vi "readfile.vi"(9 "count":i32=-1, 10 "file (use dialog)":path) -> (0 "channels":dbl[][](array[numeric]), 1 "clipping":dbl[][](array[numeric]), 2 "attenuator":dbl[][](array[numeric]), 3 "voltage":dbl[](array[numeric]), 4 "XY Graph":cluster{dbl[], dbl[]}[](graph), 6 "XY Graph 2":cluster{dbl[], dbl[]}[](graph))   [LabVIEW 2009]
panel:
  in  "file out":string="all"
  in  "file":string="all"
  out "element":i32
  out "Numeric 3":i32
  out "Numeric 2":i32
  out "size(s)":i32[](array[numeric])
  out "subarray 2":dbl[](array[numeric])
  out "Data":dbl[][][](array[numeric])
  out "data":dbl[][](array[numeric])
  out "clipping array":dbl[](array[numeric])
  out "attenuator array":dbl[](array[numeric])
  out "channels array":dbl[](array[numeric])
  out "before substring":string
  out "Numeric":i32
  out "length":i32
  out "cancelled":bool
  in  "prompt (Open existing file)":string
  out "refnum out":refnum<file>
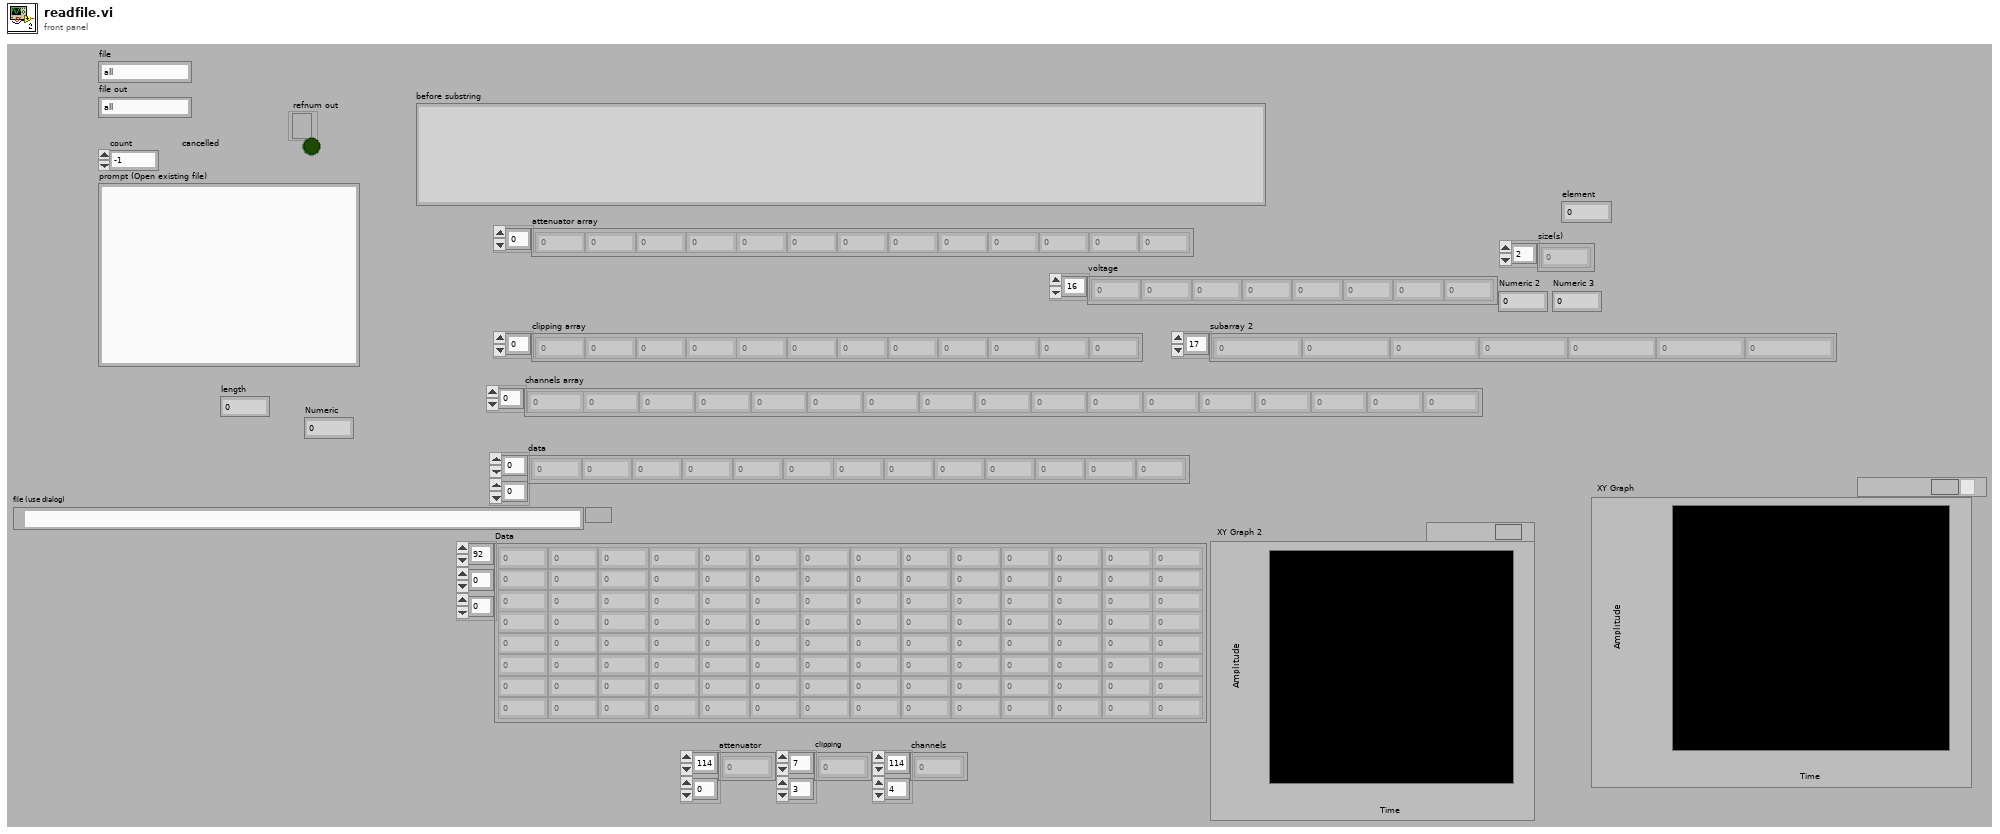
[diagram p1: front panel]
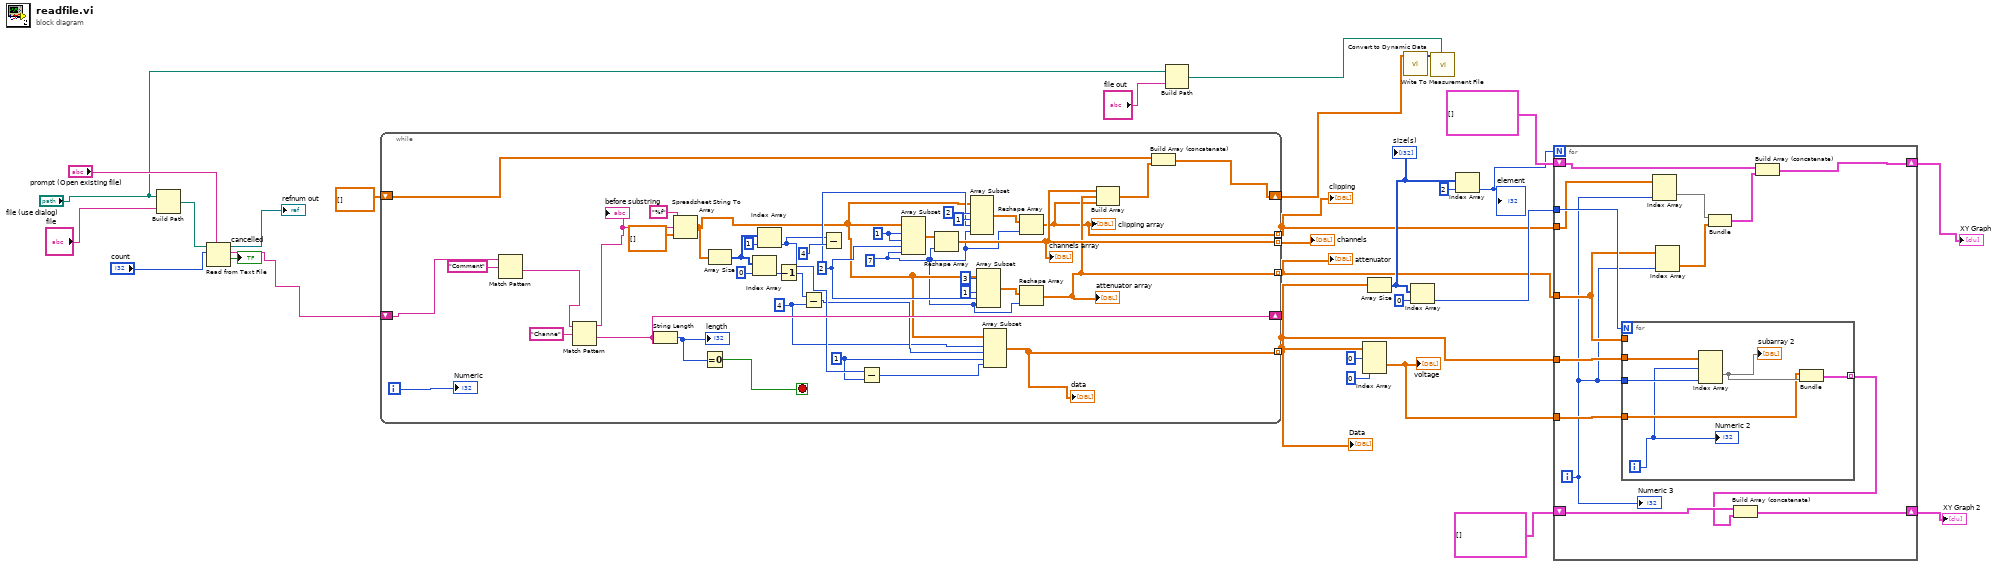
[diagram p0: block diagram]
diagram:
  n1 = Build Path(base path="file (use dialog)", name or relative path="file") -> (appended path=w6:path)
  n2 = Read from Text File(prompt (Open existing file)="prompt (Open existing file)", file (use dialog)=w6, count="count") -> (refnum out=→"refnum out":refnum<file>, text=w25:string, cancelled=→"cancelled":bool)  [unwired: 1 in, 1 out]
  n3 = while {
    shift-right: [w63] -> _
    shift-left: w25 -> [w66]
    tunnel: [w34] -> w9 mode=indexing
    tunnel: [w36] -> w11 mode=indexing
    tunnel: [w37] -> w12 mode=indexing
    tunnel: [w35] -> w10 mode=indexing
    shift-right: [w32] -> w2
    shift-left: dbl[][] [] -> [w31]
    i -> [w67]
    stop <- w68 stop-if-true
    w30 = 7 ("y")
    w38 = 1 ("index")
    w40 = 4 ("y")
    w55 = 1 ("length")
    w52 = 2 ("index")
    n4 = Match Pattern(string=w66, regular expression="Comment") -> (after substring=w64:string)  [unwired: 1 in, 3 out]
    n5 = Match Pattern(string=w64, regular expression="Channe") -> (before substring=w61:string, after substring=w63:string)  [unwired: 1 in, 2 out]
    "before substring" <- w61
    n6 = String Length(string=w63) -> (length=w69:i32)
    "length" <- w69
    n7 = Spreadsheet String To Array(format string="%f", spreadsheet string=w61, array type (2D Dbl)=dbl[][] []) -> (array=w42:dbl[][])  [unwired: 1 in]
    n8 = Equal To 0?(x=w69) -> (x = 0?=w68:bool)
    n9 = Array Size(array=w42) -> (size(s)=w47:i32[])
    n10 = Index Array(array=w47, index=0) -> (element=w44:i32)
    n11 = Index Array(array=w47, index=1) -> (element=w45:i32)
    n12 = Decrement(x=w44) -> (x-1=w43:i32)
    n13 = Subtract(x=w43, y=w40) -> (x-y=w41:i32)
    n14 = Subtract(x=w45, y=4) -> ()  [unwired: 1 out]
    n15 = Subtract(x=w45, y=w38) -> (x-y=w39:i32)
    n16 = Array Subset(array=w42, index (row)=w55, length (row)=w55, index (col)=w52, length (col)=w30) -> (w58:dbl[][])
    n17 = Reshape Array(w58, w30) -> (w36:dbl[])
    "channels array" <- w36
    n18 = Array Subset(array=w42, index (row)=2 ("index"), length (row)=1 ("length"), index (col)=w52, length (col)=w30) -> (w49:dbl[][])
    n19 = Array Subset(array=w42, index (row)=3 ("index"), length (row)=1 ("length"), index (col)=w52, length (col)=w30) -> (w48:dbl[][])
    n20 = Array Subset(array=w42, index (row)=w40, length (row)=w41, index (col)=w38, length (col)=w39) -> (w37:dbl[][])
    "data" <- w37
    n21 = Reshape Array(w49, w30) -> (w34:dbl[])
    "clipping array" <- w34
    n22 = Reshape Array(w48, w30) -> (w35:dbl[])
    "attenuator array" <- w35
    n23 = Build Array(w36, w35, w34) -> (w33:dbl[][])
    n24 = Build Array (concatenate)(w31, w33) -> (w32:dbl[][])
    "Numeric" <- w67
  }
  "Data" <- w12
  "attenuator" <- w10
  "clipping" <- w9
  "channels" <- w11
  n25 = Build Path(base path="file (use dialog)", name or relative path="file out") -> (appended path=w3:path)
  n26 = Index Array(array=w12, index (dim 0)=0 ("disabled index (page)"), index (dim 2)=0 ("disabled index (col)")) -> (element=w22:dbl[])  [unwired: 1 in]
  "voltage" <- w22
  n27 = Array Size(array=w12) -> (size(s)=w19:i32[])
  "size(s)" <- w19
  n28 = call "Convert to Dynamic Data"("2D Array"=w2) -> ("Dynamic Data Type"=w8:dynamicdata)  [unwired: 3 in]
  n29 = Index Array(array=w19, index=0) -> (element=w21:i32)
  n30 = call "Write To Measurement File"("Signals"=w8, "Filename"=w3) -> ()  [unwired: 15 in, 3 out]
  n31 = Index Array(array=w19, index=2) -> (element=w13:i32)
  "element" <- w13
  n32 = for {
    N: w13 -> [_]
    tunnel: w22 -> [w83]
    tunnel: w12 -> [w82]
    tunnel: w21 -> [w76]
    tunnel: w9 -> [w75]
    tunnel: w10 -> [w74]
    shift-right: [w80] -> w16
    shift-left: cluster{dbl[], dbl[]}[] [] ("array") -> [w81]
    shift-right: [w79] -> w15
    shift-left: cluster{dbl[], dbl[]}[] [] ("array") -> [w78]
    i -> [w70]
    n33 = for {
      N: w76 -> [_]
      tunnel: w82 -> [w89]
      tunnel: w83 -> [w87]
      tunnel: [w86] -> w77 mode=indexing
      tunnel: w74 -> [_]
      tunnel: w70 -> [w85]
      i -> [w84]
      n34 = Index Array(array=w89, index (dim 0)=w84, index (dim 2)=w85) -> (element=w88:dbl[])  [unwired: 1 in]
      "subarray 2" <- w88
      n35 = Bundle(w87, w88) -> (w86:cluster{dbl[], dbl[]})  [unwired: 1 in]
      "Numeric 2" <- w84
    }
    n36 = Index Array(array=w75, index (col)=w70) -> (element=w73:dbl[])  [unwired: 1 in]
    n37 = Index Array(array=w74, index (col)=w70) -> (element=w72:dbl[])  [unwired: 1 in]
    n38 = Bundle(w73, w72) -> (w71:cluster{dbl[], dbl[]})  [unwired: 1 in]
    n39 = Build Array (concatenate)(w78, w77) -> (w79:cluster{dbl[], dbl[]}[])
    n40 = Build Array (concatenate)(w81, w71) -> (w80:cluster{dbl[], dbl[]}[])
    "Numeric 3" <- w70
  }
  "XY Graph 2" <- w15
  "XY Graph" <- w16
